vi "set_settings_cluster.vi"(8 "error in (no error)":errorcluster, 10 "settings cluster variant":variant, 11 "StimulatorDL090503 in":refnum<class "StimulatorDL090503.lvclass">) -> (0 "error out":errorcluster, 3 "StimulatorDL090503 out":refnum<class "StimulatorDL090503.lvclass">)   [LabVIEW 2010, in "StimulatorDL090503.lvclass"]
uses:
  StimulatorDL090503.lvclass
  StimulatorDL090503.lvclass/StimulatorDL090503.ctl
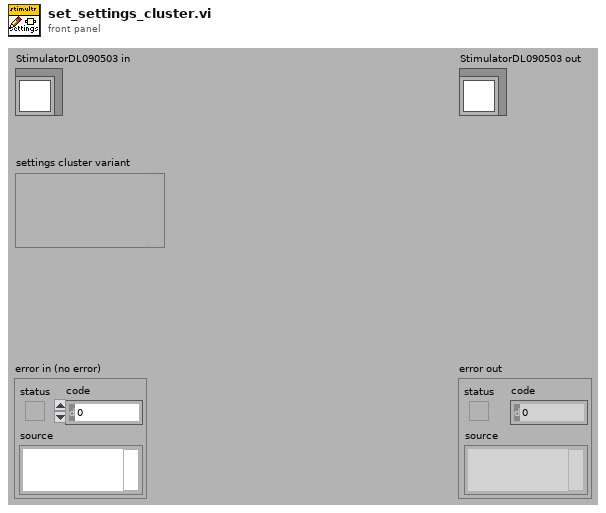
[diagram p1: front panel]
types:
  T1 = typedef "StimulatorDL090503.lvclass/settings_cluster.ctl" = cluster{"application parameters":T2, "pattern":T3}
  T2 = typedef "StimulatorDL090503Scaffold.lvclass/stimulus_application_parameters_cluster.ctl" = cluster{"duration":dbl[unit], "offset":dbl[unit], "repetition period":dbl[unit], "repetitions":i32}
  T3 = typedef "StimulatorDL090503.lvclass/pattern_parameters_cluster.ctl" = cluster{"pattern":T4, "frequency":dbl[unit], "amplitude":dbl, "offset":dbl}
  T4 = typedef "StimulatorDL090503.lvclass/pattern_type_enum.ctl" = enum16{"sine", "square (+/-)", "square (+)", "square (-)"}
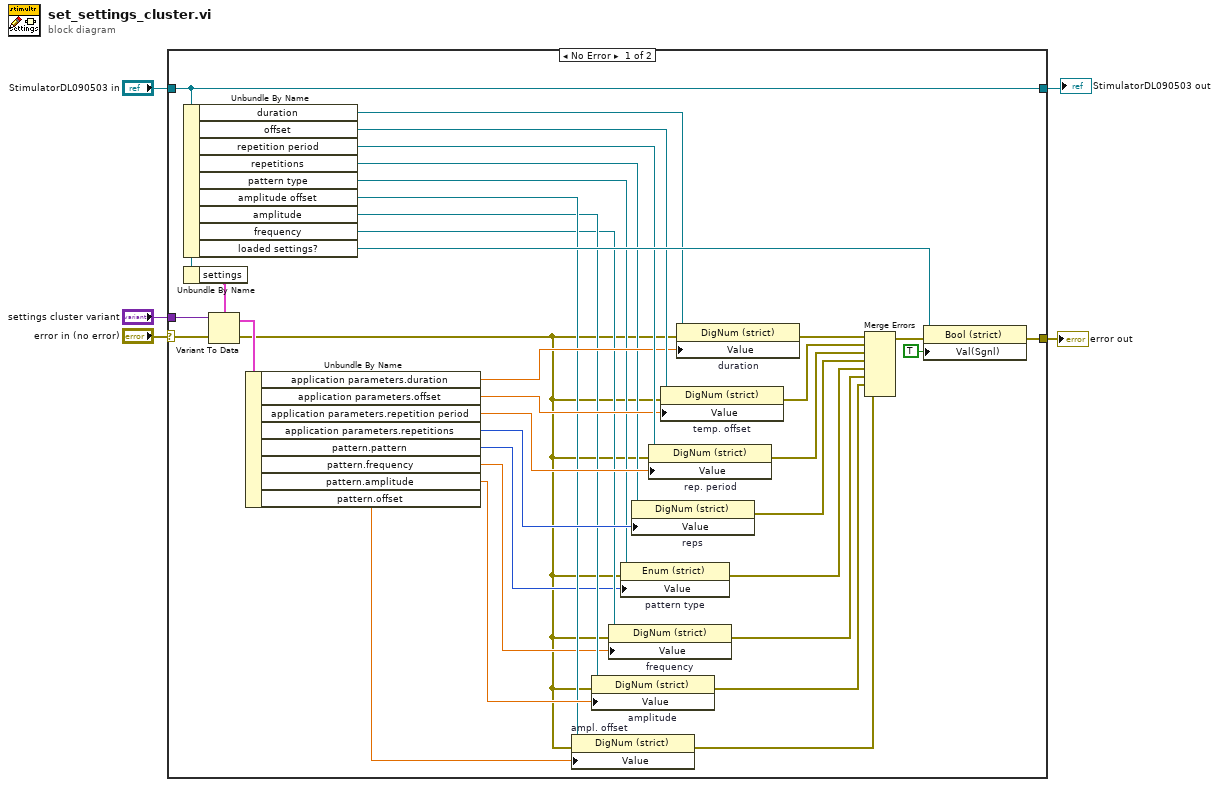
[diagram p0: block diagram]
diagram:
  n1 = case shown="No Error" "error in (no error)" {
    selector: "error in (no error)" -> [w39 w40]
    tunnel: "settings cluster variant" -> [w38 _]
    tunnel: "StimulatorDL090503 in" -> [w35 w41]
    tunnel: [w32 w40] -> w2
    tunnel: [w35 w41] -> w1
    frame No Error {
      n2 = Unbundle By Name(w35) -> ("duration"=w31:refnum<vi>, "offset"=w30:refnum<vi>, "repetition period"=w29:refnum<vi>, "repetitions"=w25:refnum<vi>, "pattern type"=w18:refnum<vi>, "amplitude offset"=w15:refnum<vi>, "amplitude"=w14:refnum<vi>, "frequency"=w13:refnum<vi>, "loaded settings?"=w34:refnum<vi>)
      n3 = Unbundle By Name(w35) -> ("settings"=w37:T1)
      n4 = Variant To Data(error in=w39, Variant=w38, type=w37) -> (error out=w6:errorcluster, data=w36:T1)
      n5 = Unbundle By Name(w36) -> ("application parameters.duration"=w28:dbl[unit], "application parameters.offset"=w27:dbl[unit], "application parameters.repetition period"=w26:dbl[unit], "application parameters.repetitions"=w24:i32, "pattern.pattern"=w8:T4, "pattern.frequency"=w7:dbl[unit], "pattern.amplitude"=w16:dbl, "pattern.offset"=w17:dbl)
      n6 = property on="ampl. offset" class="DigNum (strict)"(reference=w15, error in=w6, "Value"=w17) -> (error out=w9:errorcluster)  [unwired: 1 out]
      n7 = property on="amplitude" class="DigNum (strict)"(reference=w14, error in=w6, "Value"=w16) -> (error out=w10:errorcluster)  [unwired: 1 out]
      n8 = property on="frequency" class="DigNum (strict)"(reference=w13, error in=w6, "Value"=w7) -> (error out=w11:errorcluster)  [unwired: 1 out]
      n9 = property on="pattern type" class="Enum (strict)"(reference=w18, error in=w6, "Value"=w8) -> (error out=w12:errorcluster)  [unwired: 1 out]
      n10 = property on="reps" class="DigNum (strict)"(reference=w25, "Value"=w24) -> (error out=w20:errorcluster)  [unwired: 1 in, 1 out]
      n11 = property on="rep. period" class="DigNum (strict)"(reference=w29, error in=w6, "Value"=w26) -> (error out=w21:errorcluster)  [unwired: 1 out]
      n12 = property on="temp. offset" class="DigNum (strict)"(reference=w30, error in=w6, "Value"=w27) -> (error out=w22:errorcluster)  [unwired: 1 out]
      n13 = property on="duration" class="DigNum (strict)"(reference=w31, error in=w6, "Value"=w28) -> (error out=w23:errorcluster)  [unwired: 1 out]
      n14 = Merge Errors(w23, w22, w21, w20, w12, w11, w10, w9) -> (w19:errorcluster)
      n15 = property class="Bool (strict)"(reference=w34, error in=w19, "Val(Sgnl)"=TRUE ("Value (Signaling)")) -> (error out=w32:errorcluster)  [unwired: 1 out]
    }
    frame Error {
    }
  }
  "error out" <- w2
  "StimulatorDL090503 out" <- w1
